vi "Write Unique Test ID.vi"(10 "Unique Test ID":string, 11 "Assert":refnum<class "Assert.lvclass">) -> (3 "Assert out":refnum<class "Assert.lvclass">)   [LabVIEW 2020, in "Caraya.lvlib" / "Assert.lvclass"]
uses:
  Assert.lvclass
  Assert.lvclass/Assert.ctl
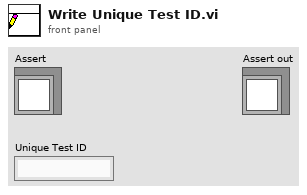
[diagram p1: front panel]
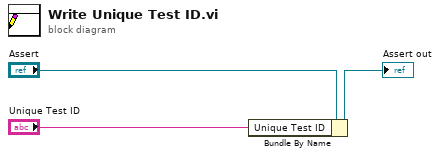
[diagram p0: block diagram]
diagram:
  n1 = Bundle By Name(cluster="Assert", "Unique Test ID"="Unique Test ID") -> (→"Assert out":refnum<class "Assert.lvclass">)
